vi "CtlsReplaceFailed.vi"() -> ()   [LabVIEW 2016, in "SwitchDependenciesVariables.lvlib"]
uses:
  SwitchDependenciesVariables.lvlib
panel:
  in  "CtlsReplaceFailed":string
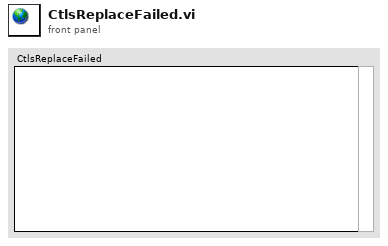
[diagram p1: front panel]
diagram:
